vi "StartTimerEngineThread.vi"(8 "error in (no error)":errorcluster, 11 "DVR":refnum<data-value>) -> (0 "error out":errorcluster)   [LabVIEW 2017, in "TimerEngine.lvlib" / "TimerEngine.lvclass"]
uses:
  TimerEngine.lvclass
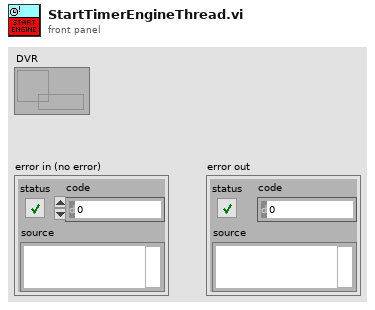
[diagram p1: front panel]
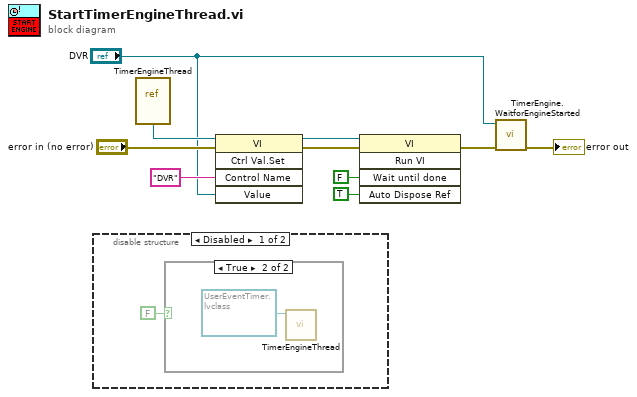
[diagram p0: block diagram]
diagram:
  n1 = disable-structure shown="Disabled" {
    frame Disabled {
      n2 = case shown="True" FALSE {
        frame False {
        }
        frame True {
          n3 = call "TimerEngineThread.vi"("DVR"=refnum<data-value> refnum) -> ()  [unwired: 11 in]
        }
      }
    }
    frame Enabled {
    }
  }
  n4 = vi-ref "TimerEngineThread.vi"() -> (w7:refnum<vi>)
  n5 = invoke class="VI" method="Ctrl Val.Set"(reference=w7, error in="error in (no error)", "Control Name"="DVR", "Value"="DVR") -> (reference out=w5:refnum<vi>, error out=w3:errorcluster)  [unwired: 1 in, 3 out]
  n6 = invoke class="VI" method="Run VI"(reference=w5, error in=w3, "Wait until done"=FALSE ("Wait Until Done"), "Auto Dispose Ref"=TRUE ("Auto Dispose Reference")) -> (error out=w10:errorcluster)  [unwired: 1 in, 4 out]
  n7 = call "TimerEngine.WaitforEngineStarted.vi"("error in (no error)"=w10, "DVR"="DVR") -> ("error out"=→"error out":errorcluster)  [unwired: 8 in, 1 out]
